vi "Set Timestamp Day of the Week.vi"(2 "Weekly DoW":T1 caption="DoW", 3 "Time Stamp":timestamp) -> (1 "Time Stamp out":timestamp)   [LabVIEW 2020, in "ARecurrence.lvclass"]
uses:
  ARecurrence.lvclass
  Day of the Week STYP.ctl
  ARecurrence.lvclass/ARecurrence.ctl
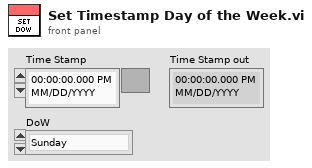
[diagram p1: front panel]
types:
  T1 = typedef "Day of the Week STYP.ctl" = enum16{"Sunday", "Monday", "Tuesday", "Wednesday", "Thursday", "Friday", "Saturday"}
  T2 = typedef "LVDateTimeRec.ctl" = cluster{"fractional second":dbl, "second":i32, "minute":i32, "hour":i32, "day of month":i32, "month":i32, "year":i32, "day of week":i32, "day of year":i32, "DST":i32}
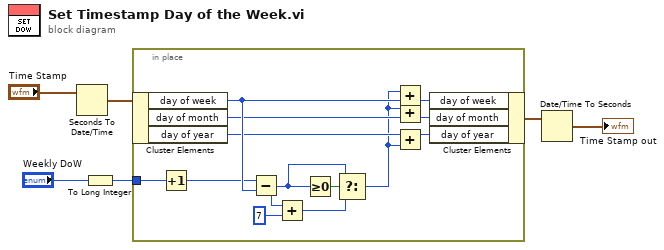
[diagram p0: block diagram]
diagram:
  n1 = Seconds To Date/Time(time stamp (now)="Time Stamp") -> (date time rec=w6:T2)  [unwired: 1 in]
  n2 = To Long Integer(number="Weekly DoW") -> (32bit integer=w1:i32)
  n3 = in-place {
    in-place-border: w1 -> [w18]
    n4 = in-place-cluster #1(w6) -> ("day of week"=w17:i32, "day of month"=w16:i32, "day of year"=w15:i32)
    n5 = Increment(x=w18) -> (x+1=w11:i32)
    n6 = Subtract(x=w11, y=w17) -> (x-y=w8:i32)
    n7 = Add(x=w8, y=7) -> (x+y=w9:i32)
    n8 = Greater Or Equal To 0?(x=w8) -> (x >= 0?=w10:bool)
    n9 = Select(t=w8, s=w10, f=w9) -> (s? t:f=w7:i32)
    n10 = Add(x=w7, y=w17) -> (x+y=w14:i32)
    n11 = Add(x=w7, y=w16) -> (x+y=w13:i32)
    n12 = Add(x=w15, y=w7) -> (x+y=w12:i32)
    n13 = in-place-cluster #1("day of week"=w14, "day of month"=w13, "day of year"=w12) -> (w4:T2)
  }
  n14 = Date/Time To Seconds(2:w4) -> (0:→"Time Stamp out":timestamp)  [unwired: 1 in]
